vi "iXonRTA.vi"() -> ()   [LabVIEW 2009]
panel:
  out "Acquiring":bool
  out "Intensity Graph":i32[][](graph)
  out "SetTriggerMode":u32
  out "SetVSSpeed":u32
  out "SetHSSpeed":u32
  out "GetMostRecentImage":u32
  out "Image Array":i32[](array[numeric]) caption="Array"
  in  "stop":bool
  out "Shutdown":u32
  out "GetDetector":u32
  out "Y Pixels":i32
  out "Total number of pixels":i32
  out "SetImage":u32
  out "X Pixels":i32
  out "SetExposureTime":u32
  out "SetReadMode":u32
  out "SetAcquisition Mode":u32
  out "Start Acquisition":u32
  in  "Exposure Time (secs)":sgl=0.1 format="%.2f"
  out "Initialize":u32
  # "INPUT"
  # "Return Values"
  # "Numerical data"
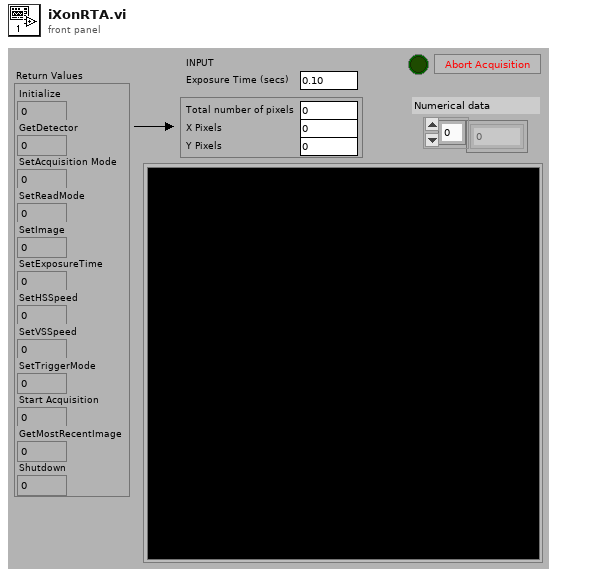
[diagram p1: front panel]
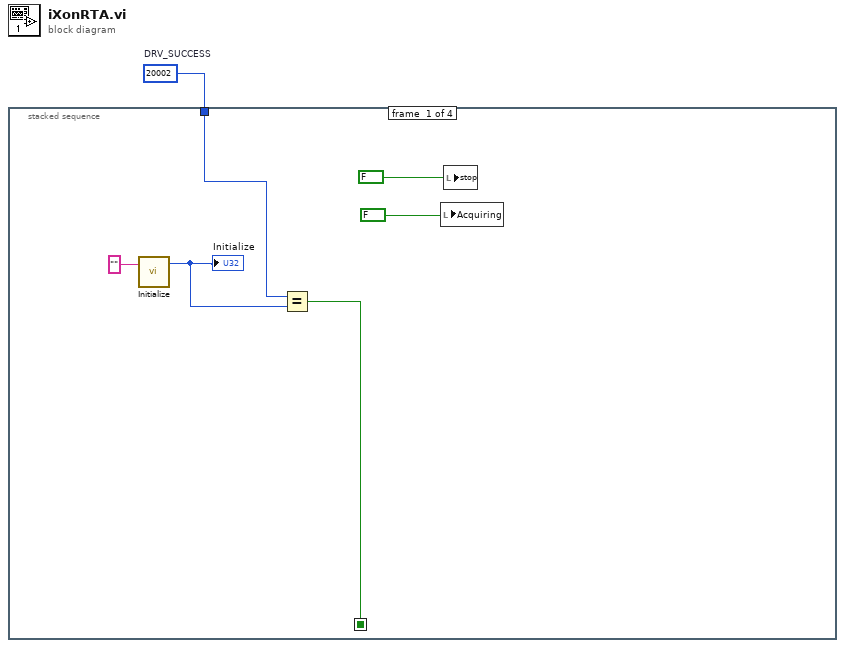
[diagram p0: block diagram]
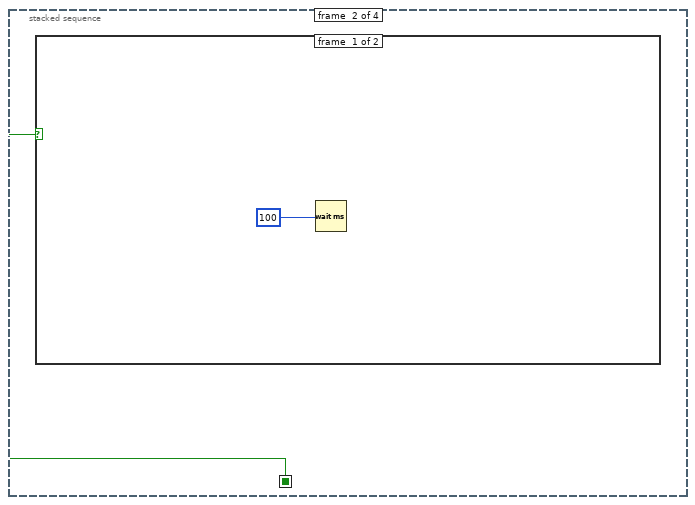
[diagram p2: hidden frame]
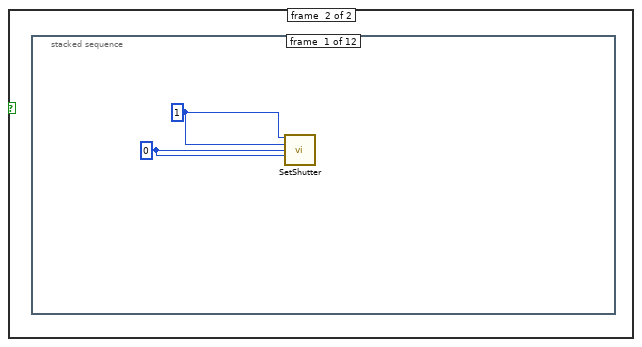
[diagram p3: hidden frame]
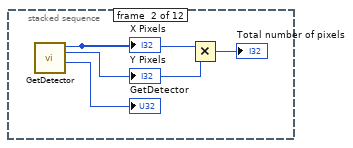
[diagram p4: hidden frame]
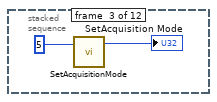
[diagram p5: hidden frame]
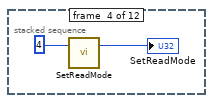
[diagram p6: hidden frame]
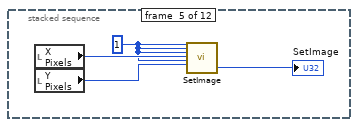
[diagram p7: hidden frame]
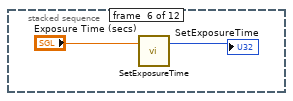
[diagram p8: hidden frame]
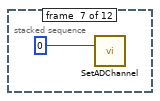
[diagram p9: hidden frame]
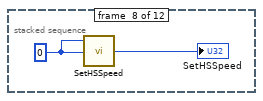
[diagram p10: hidden frame]
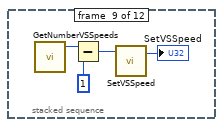
[diagram p11: hidden frame]
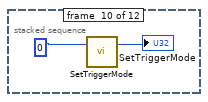
[diagram p12: hidden frame]
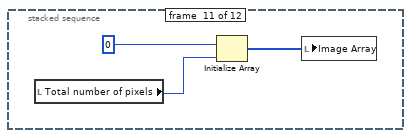
[diagram p13: hidden frame]
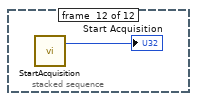
[diagram p14: hidden frame]
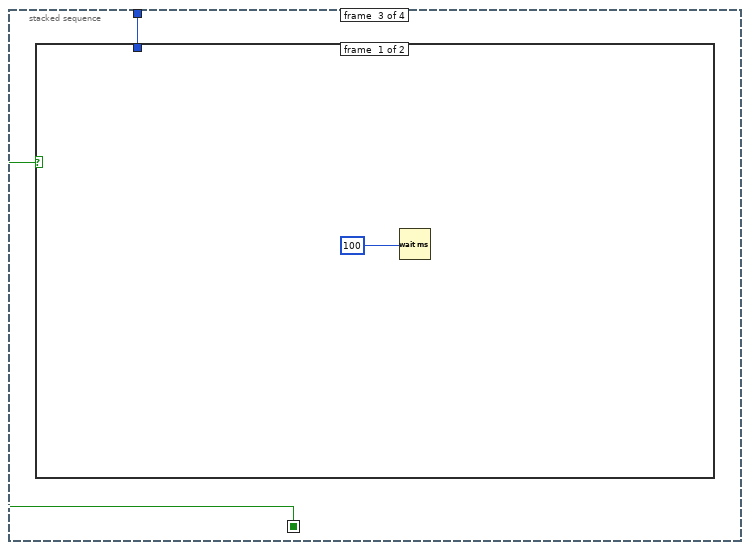
[diagram p15: hidden frame]
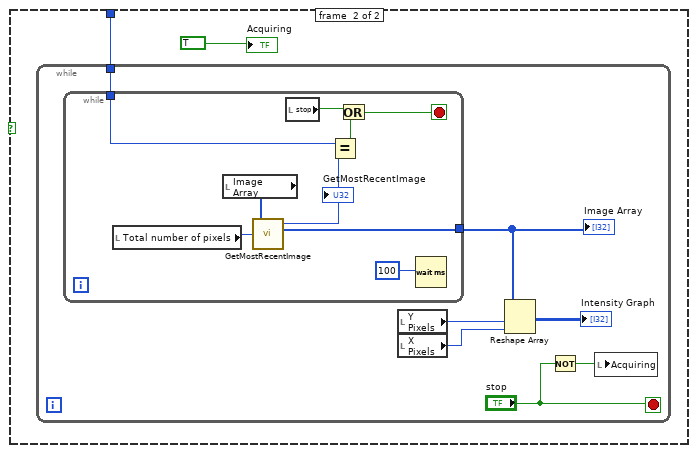
[diagram p16: hidden frame]
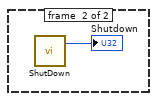
[diagram p18: hidden frame]
diagram:
  w1 = 20002  # DRV_SUCCESS
  n1 = stacked-sequence {
    seq-local: [w6 _ _ _] -> [_ w8 w40 w60]
    tunnel: w1 -> [w7 _ w39 _]
    frame #0 {
      n2 = call <userlib>:"Initialize.vi"("directory (\"\")"="") -> ("DLL error code"=w2:u32)  [unwired: 1 in, 1 out]
      "Initialize" <- w2
      n3 = Equal?(x=w7, y=w2) -> (x = y?=w6:bool)
      n4 = local write "Acquiring"(FALSE) -> ()
      n5 = local write "stop"(FALSE) -> ()
    }
    frame #1 {
      n6 = case shown="True" w8 {
        frame #0 {
          n7 = Wait (ms)(milliseconds to wait=100) -> ()  [unwired: 1 out]
        }
        frame #1 {
          n8 = stacked-sequence {
            frame #0 {
              w11 = 1
              w10 = 0
              n9 = call <userlib>:"SetShutter.vi"("type"=w11, "mode"=w11, "closingtime"=w10, "openingtime"=w10) -> ()  [unwired: 10 in, 2 out]
            }
            frame #1 {
              n10 = call <userlib>:"GetDetector.vi"() -> ("DLL error code"=→"GetDetector":u32, "ypixels"=w14:i32, "xpixels"=w13:i32)  [unwired: 4 in, 1 out]
              "X Pixels" <- w13
              "Y Pixels" <- w14
              n11 = Multiply(x=w13, y=w14) -> (x*y=→"Total number of pixels":i32)
            }
            frame #2 {
              n12 = call <userlib>:"SetAcquisitionMode.vi"("mode"=u16 5 ("AcquisitionMode")) -> ("DLL error code"=→"SetAcquisition Mode":u32)  [unwired: 1 in, 1 out]
            }
            frame #3 {
              n13 = call <userlib>:"SetReadMode.vi"("mode"=u16 4 ("ReadMode")) -> ("DLL error code"=→"SetReadMode":u32)  [unwired: 1 in, 1 out]
            }
            frame #4 {
              w22 = 1
              n14 = local read "X Pixels"() -> (w23:i32)
              n15 = local read "Y Pixels"() -> (w21:i32)
              n16 = call <userlib>:"SetImage.vi"("hbin"=w22, "vbin"=w22, "hstart"=w22, "hend"=w23, "vstart"=w22, "vend"=w21) -> ("DLL error code"=→"SetImage":u32)  [unwired: 20 in, 1 out]
            }
            frame #5 {
              n17 = call <userlib>:"SetExposureTime.vi"("time"="Exposure Time (secs)") -> ("DLL error code"=→"SetExposureTime":u32)  [unwired: 1 in, 1 out]
            }
            frame #6 {
              n18 = call <userlib>:"SetADChannel.vi"("channel"=0) -> ()  [unwired: 1 in, 2 out]
            }
            frame #7 {
              w27 = 0 ("input param")
              n19 = call <userlib>:"SetHSSpeed.vi"("index"=w27, "type"=w27) -> ("DLL error code"=→"SetHSSpeed":u32)  [unwired: 2 in, 1 out]
            }
            frame #8 {
              n20 = call <userlib>:"GetNumberVSSpeeds.vi"() -> ("number"=w31:i32)  [unwired: 3 in, 2 out]
              n21 = Subtract(x=w31, y=1) -> (x-y=w29:i32)
              n22 = call <userlib>:"SetVSSpeed.vi"("index"=w29) -> ("DLL error code"=→"SetVSSpeed":u32)  [unwired: 1 in, 1 out]
            }
            frame #9 {
              n23 = call <userlib>:"SetTriggerMode.vi"("mode"=0) -> ("DLL error code"=→"SetTriggerMode":u32)  [unwired: 1 in, 1 out]
            }
            frame #10 {
              n24 = local read "Total number of pixels"() -> (w36:i32)
              n25 = Initialize Array(0, w36) -> (w35:i32[])
              n26 = local write "Image Array"(w35) -> ()
            }
            frame #11 {
              n27 = call <userlib>:"StartAcquisition.vi"() -> ("DLL error code"=→"Start Acquisition":u32)  [unwired: 2 in, 1 out]
            }
          }
        }
      }
    }
    frame #2 {
      n28 = case shown="True" w40 {
        tunnel: w39 -> [_ w43]
        frame #0 {
          n29 = Wait (ms)(milliseconds to wait=100) -> ()  [unwired: 1 out]
        }
        frame #1 {
          n30 = while {
            tunnel: w43 -> [w44]
            stop <- "stop" stop-if-true
            n31 = while {
              tunnel: [w55] -> w50
              tunnel: w44 -> [w52]
              stop <- w58 stop-if-true
              n32 = local read "Total number of pixels"() -> (w57:i32)
              n33 = local read "Image Array"() -> (w56:i32[])
              n34 = call <userlib>:"GetMostRecentImage.vi"("size"=w57, "array"=w56) -> ("array"=w55:i32[], "DLL error code"=w53:u32)  [unwired: 1 in, 1 out]
              "GetMostRecentImage" <- w53
              n35 = local read "stop"() -> (w54:bool)
              n36 = Equal?(x=w52, y=w53) -> (x = y?=w51:bool)
              n37 = Or(x=w54, y=w51) -> (x .or. y?=w58:bool)
              n38 = Wait (ms)(milliseconds to wait=100) -> ()  [unwired: 1 out]
            }
            "Image Array" <- w50
            n39 = local read "Y Pixels"() -> (w48:i32)
            n40 = local read "X Pixels"() -> (w47:i32)
            n41 = Reshape Array(w50, w48, w47) -> (→"Intensity Graph":i32[][])
            n42 = Not(x="stop") -> (.not. x?=w46:bool)
            n43 = local write "Acquiring"(w46) -> ()
          }
          "Acquiring" <- TRUE
        }
      }
    }
    frame #3 {
      n44 = case shown="True" w60 {
        frame #0 {
        }
        frame #1 {
          n45 = call <userlib>:"ShutDown.vi"() -> ("DLL error code"=→"Shutdown":u32)  [unwired: 2 in, 1 out]
        }
      }
    }
  }
